vi "Global1.vi"() -> ()   [LabVIEW 2012]
panel:
  in  "SQLM100dsn":path=path "c:/m100/data/m100.dsn"
  in  "PathHotLotReportXlsOutput":path=path "o:/monitor/hotlot.xls"
  in  "PathHotLotReportXlsTemplate":path=path "c:/m100/data/hotlot.xls"
  in  "PathHotLot":path=path "o:/monitor/hotLot"
  in  "PathDailyReportOutput":path=path "o:/monitor"
  in  "PathDailyReportXlsTemplate":path=path "c:/m100/data/at.xls"
  in  "PathMonitorXlsOutput":path=path "o:/monitor/monitor1.xls"
  in  "PathMonitorXlsTemplete":path=path "c:/m100/data/monitor.xls"
  in  "PathMcsUdl":path=path "c:/m100/data/mcs.udl"
  in  "PathM100Log":path=path "c:/m100/log"
  in  "PathM100":path=path "c:/m100"
  in  "PathM100dsn":path=path "c:/m100/data/m1003.dsn"
  out "PathEntity":path=path "c:/m100/data/entity.txt"
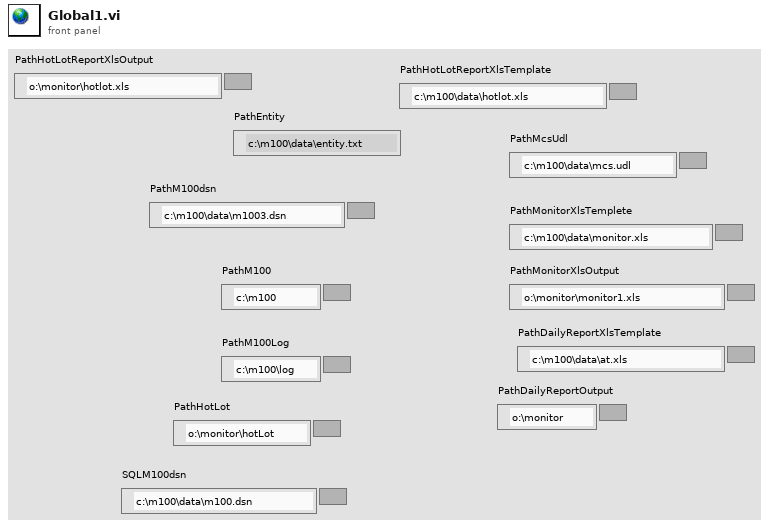
[diagram p1: front panel]
diagram:
